vi "UpdatePositionInfoControl.vi"(9 "ImageInfo":T1, 10 "Y":refnum<vi>, 11 "Digital in":refnum<vi>) -> ()   [LabVIEW 2017]
uses:
  Types/ImageInfo.ctl
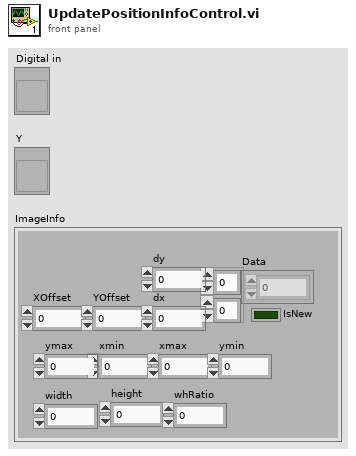
[diagram p1: front panel]
types:
  T1 = typedef "ImageInfo.ctl" = cluster{"IsNew":bool, "Data":dbl[][], "XOffset":dbl, "YOffset":dbl, "dy":dbl, "dx":dbl, "xmin":dbl, "xmax":dbl, "ymin":dbl, "ymax":dbl, "width":dbl, "height":dbl, "whRatio":dbl}
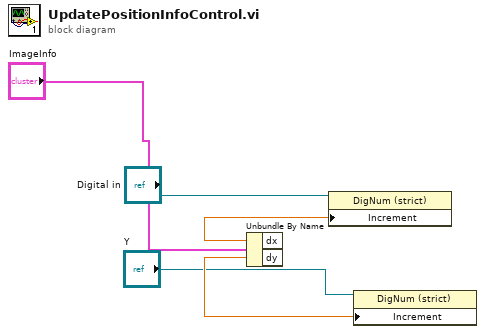
[diagram p0: block diagram]
diagram:
  n1 = Unbundle By Name("ImageInfo") -> ("dx"=w3:dbl, "dy"=w5:dbl)
  n2 = property class="DigNum (strict)"(reference="Digital in", "Increment"=w3) -> ()  [unwired: 1 in, 2 out]
  n3 = property class="DigNum (strict)"(reference="Y", "Increment"=w5) -> ()  [unwired: 1 in, 2 out]
